vi "LEP_RV_MemoryMap.vi"() -> ()   [LabVIEW 2011]
doc: "Define memory mapping for the Axiom CMD565 target."
uses:
  <vilib>/LabVIEW Targets/Embedded/Utilities/MemMap/EMB_Utility_MemMap_VI_Compare.ctl
  <vilib>/LabVIEW Targets/Embedded/Utilities/MemMap/EMB_Utility_MemMap_VI_Default.ctl
  <vilib>/LabVIEW Targets/Embedded/Utilities/MemMap/EMB_Utility_MemMap_VI_Config.ctl
  <vilib>/LabVIEW Targets/Embedded/Utilities/MemMap/EMB_Utility_MemMap_VI_Type.ctl
  <vilib>/Platform/EmbProject/Plugins/utilities/LEP_Utilities_GetSetProjectData_Variant.vi
panel:
  in  "Default Config":T1
  in  "Compare":T2
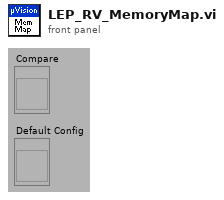
[diagram p1: front panel]
types:
  T1 = typedef "EMB_Utility_MemMap_VI_Default.ctl" = refnum<vi>
  T2 = typedef "EMB_Utility_MemMap_VI_Compare.ctl" = refnum<vi>
  T3 = typedef "EMB_Utility_MemMap_VI_Config.ctl" = cluster{"filename":string, "Code Section":i32, "Code Section List":i32[], "Const Section":i32, "Const Section List":i32[], "VI Type":T4}
  T4 = typedef "EMB_Utility_MemMap_VI_Type.ctl" = enum32{"invalid VI type", "Standard VI", "Control VI", "Global VI", "Polymorphic VI", "Configuration VI", "SubSystem"}
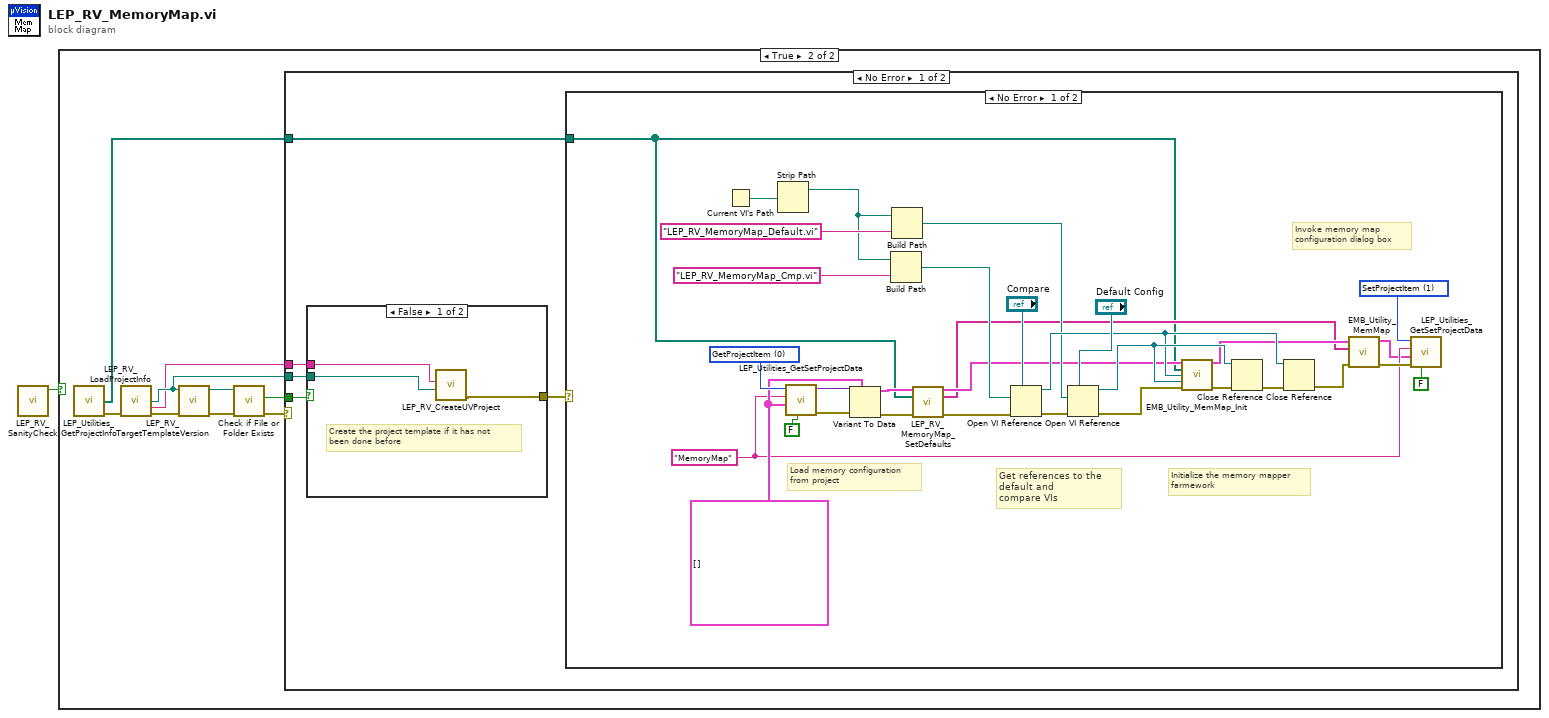
[diagram p0: block diagram]
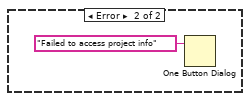
[diagram p5: hidden frame]
diagram:
  n1 = call "LEP_RV_SanityCheck.vi"() -> ("ok"=w1:bool)  [unwired: 10 in, 1 out]
  n2 = case shown="True" w1 {
    frame False {
    }
    frame True {
      n3 = call <vilib>:"LEP_Utilities_GetProjectInfo.vi"() -> ("SourceFiles"=w6:path[], "error out"=w7:errorcluster)  [unwired: 11 in, 3 out]
      n4 = call "LEP_RV_LoadProjectInfo.vi"("error in (no error)"=w7) -> ("Build Path"=w3:path, "Target Name"=w2:string, "error out"=w10:errorcluster)  [unwired: 8 in, 4 out]
      n5 = call "LEP_RV_TargetTemplateVersion.vi"("error in (no error)"=w10, "Path"=w3) -> ("error out"=w9:errorcluster, "Path plus Version"=w8:path)  [unwired: 7 in, 1 out]
      n6 = call <vilib>:"Check if File or Folder Exists.vi"("error in (no error)"=w9, "path"=w8) -> ("error out"=w5:errorcluster, "file or folder exists?"=w4:bool)  [unwired: 7 in, 1 out]
      n7 = case shown="No Error" w5 {
        tunnel: w6 -> [w15 _]
        tunnel: w4 -> [w14 _]
        tunnel: w3 -> [w12 _]
        tunnel: w2 -> [w11 _]
        frame No Error {
          n8 = case shown="False" w14 {
            tunnel: [w18 _] -> w13
            tunnel: w12 -> [w17 _]
            tunnel: w11 -> [w16 _]
            frame False {
              # "Create the project template if it has not\nbeen done before"
              n9 = call "LEP_RV_CreateUVProject.vi"("Build Path"=w17, "Target"=w16) -> ("error out"=w18:errorcluster)  [unwired: 9 in]
            }
            frame True {
            }
          }
          n10 = case shown="No Error" w13 {
            tunnel: w15 -> [w19 _]
            frame No Error {
              w39 = u16 1 items=["GetProjectItem", "SetProjectItem"] ("Command")
              w46 = T3[] []
              w50 = u16 0 items=["GetProjectItem", "SetProjectItem"] ("Command")
              w40 = "MemoryMap" ("ItemName")
              # "Invoke memory map \nconfiguration dialog box"
              # "Initialize the memory mapper\nfarmework"
              # "Get references to the default and\ncompare VIs"
              # "Load memory configuration\nfrom project"
              n11 = Current VI's Path() -> (path=w30:path)
              n12 = Strip Path(path=w30) -> (stripped path=w26:path)  [unwired: 1 out]
              n13 = call-poly <vilib>:"LEP_Utilities_GetSetProjectData.vi"("access target data (F)"=FALSE ("Prefix target name?"), "Variant In"=w46, "ItemName"=w40, "Command"=w50) -> ("error out"=w48:errorcluster, "Variant Out"=w47:variant)  [unwired: 5 in, 1 out]
              n14 = Variant To Data(error in=w48, type=w46, Variant=w47) -> (data=w22:T3[], error out=w24:errorcluster)
              n15 = Build Path(base path=w26, name or relative path="LEP_RV_MemoryMap_Cmp.vi") -> (appended path=w25:path)
              n16 = Build Path(base path=w26, name or relative path="LEP_RV_MemoryMap_Default.vi") -> (appended path=w28:path)
              n17 = call "LEP_RV_MemoryMap_SetDefaults.vi"("Config In"=w22, "SourceFiles"=w19, "error in (no error)"=w24) -> ("Config Out"=w21:T3[], "Section Names"=w20:string[], "error out"=w23:errorcluster)  [unwired: 10 in]
              n18 = Open VI Reference(type specifier VI Refnum (for type only)="Compare", vi path=w25, error in (no error)=w23) -> (vi reference=w33:T2, error out=w45:errorcluster)  [unwired: 3 in]
              n19 = Open VI Reference(type specifier VI Refnum (for type only)="Default Config", vi path=w28, error in (no error)=w45) -> (vi reference=w34:T1, error out=w44:errorcluster)  [unwired: 3 in]
              n20 = call <vilib>:"EMB_Utility_MemMap_Init.vi"("Config"=w21, "Source VIs"=w19, "Compare"=w33, "Default Config"=w34, "error in (no error)"=w44) -> ("Config Out"=w31:T3[], "error out"=w36:errorcluster)  [unwired: 9 in]
              n21 = Close Reference(reference=w34, error in (no error)=w36) -> (error out=w35:errorcluster)
              n22 = Close Reference(reference=w33, error in (no error)=w35) -> (error out=w32:errorcluster)
              n23 = call <vilib>:"EMB_Utility_MemMap.vi"("error in (no error)"=w32, "Section Names"=w20, "Config"=w31) -> ("error out"=w41:errorcluster, "Config Out"=w38:T3[])  [unwired: 7 in]
              n24 = call-poly <vilib>:"LEP_Utilities_GetSetProjectData.vi"("access target data (F)"=FALSE ("Prefix target name?"), "error in"=w41, "Variant In"=w38, "ItemName"=w40, "Command"=w39) -> ()  [unwired: 4 in, 3 out]
            }
            frame Error {
            }
          }
        }
        frame Error {
          n25 = One Button Dialog(message="Failed to access project info") -> ()  [unwired: 1 in, 1 out]
        }
      }
    }
  }
